vi "Get Chamber Status-harness.vi"(11 "test case ID":string) -> (3 "result":bool)   [LabVIEW 2018]
doc: "The harness VI is executed for every test case. InstaCoverage passes the test case ID before the execution of the test case in the <b>test case ID</b> input and reads the <b>result</b> output after the execution. If the result is TRUE and no error happens during the execution, then the test case is evaluated as PASSED. If the result is false and no error happens during the execution, then the test case is evaluated as FAILED. Otherwise the test case is evaluated as ERROR.\n\nThe result of the test suite will be PASSED (FAILED) if all (at least one) test cases are PASSED (FAILED). If at least one test case in the test suite has the ERROR result, then the test suite will have ERROR result.\n\n<b>Note: </b>Don't change the connector pane of this VI.\n\nSee the Help Document for more information. (<b>Help</b> > <b>IncQuery Labs</b> > <b>InstaCoverage</b> > <b>InstaCoverage Help...</b>)"
uses:
  Libraries/Thermal Chamber Response Simulator/Thermal Chamber Response Simulator.lvlib
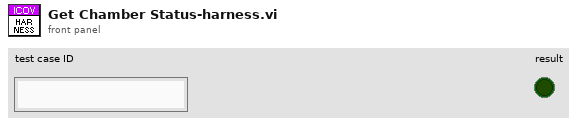
[diagram p1: front panel]
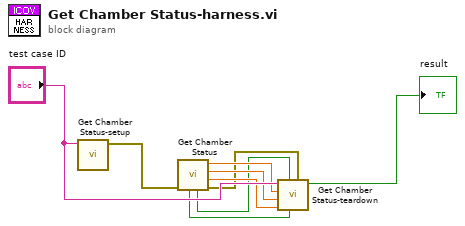
[diagram p0: block diagram]
diagram:
  n1 = call "Get Chamber Status-setup.vi"("test case ID"="test case ID") -> ("Test Error"=w2:errorcluster)  [unwired: 10 in]
  n2 = call "Get Chamber Status.vi"("error in (no error)"=w2) -> ("error out"=w1:errorcluster, "Ramp Rate (deg C / second)"=w5:dbl, "Temperature Set Point (deg C)"=w6:dbl, "Actual Temperature"=w7:dbl, "Application Exit"=w3:bool, "Heater State"=w4:bool)  [unwired: 5 in]
  n3 = call "Get Chamber Status-teardown.vi"("Test Error"=w1, "Heater State"=w4, "Application Exit"=w3, "Ramp Rate (deg C / second)"=w5, "Temperature Set Point (deg C)"=w6, "Actual Temperature"=w7, "test case ID"="test case ID") -> ("result"=→"result":bool)  [unwired: 4 in]
